vi "BRig_dataRT_stats__nReward_cur.vi"() -> (2 "output_nReward_cur":i32)   [LabVIEW 2014]
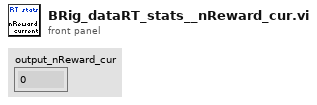
[diagram p1: front panel]
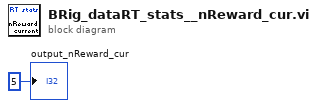
[diagram p0: block diagram]
diagram:
  "output_nReward_cur" <- 5 ("output_iBlock")
